vi "GetFeaturesForMCSA(60s).vi"(6 "supported features":string[](array[string]), 8 "error in (no error)":errorcluster, 9 "Metric Cache":variant, 11 "ChannelModel":T4) -> (0 "error out":errorcluster, 2 "channels":T1)   [LabVIEW 2017, in "McsaAnalysisFunctions.lvlib"]
uses:
  <vilib>/addons/InsightCM/Utilities/Analysis/MCSA/McsaAnalysisFunctions.lvlib
  <vilib>/addons/InsightCM/MessageBus/Base/controls/R2_Channel.ctl
  <vilib>/addons/InsightCM/MessageBus/Base/controls/KeyValuePair.ctl
  <vilib>/addons/InsightCM/MessageBus/Base/controls/Metric.ctl
  <vilib>/addons/InsightCM/Utilities/Analysis/MCSA/controls/McsaLowUpdateChannel.ctl
  <vilib>/addons/InsightCM/Utilities/Analysis/Shared/controls/Feature.ctl
  <vilib>/addons/InsightCM/Utilities/Analysis/Shared/controls/AmplitudeScale.ctl
  <vilib>/addons/InsightCM/Utilities/Analysis/Shared/AnalysisHelper.lvlib
  <vilib>/addons/InsightCM/Utilities/Tdms/Tdms.lvlib
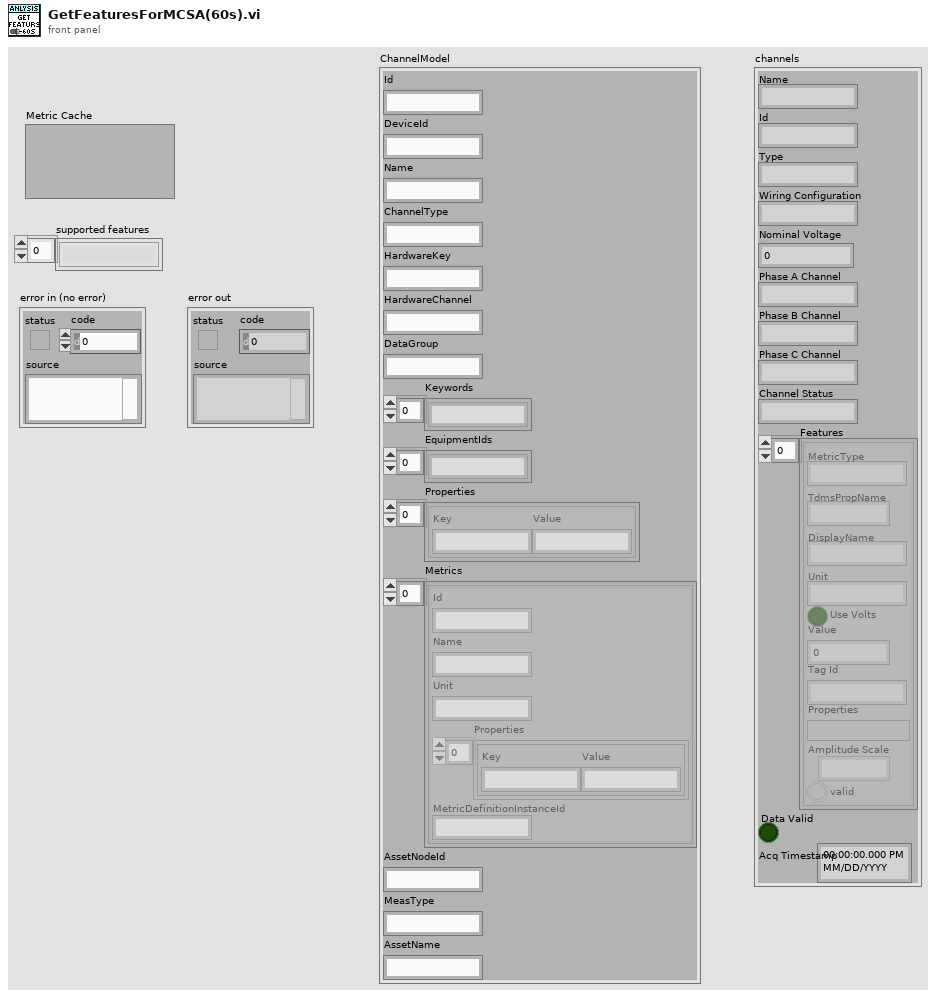
[diagram p1: front panel]
types:
  T1 = typedef "McsaAnalysisFunctions.lvlib/McsaLowUpdateChannel.ctl" = cluster{"Name":string, "Id":string, "Type":string, "Wiring Configuration":string, "Nominal Voltage":dbl, "Phase A Channel":string, "Phase B Channel":string, "Phase C Channel":string, "Channel Status":string, "Features":T2[], "Data Valid":bool, "Acq Timestamp":timestamp}
  T2 = typedef "AnalysisHelper.lvlib/Feature.ctl" = cluster{"MetricType":string, "TdmsPropName":string, "DisplayName":string, "Unit":string, "Use Volts":bool, "Value":dbl, "Tag Id":string, "Properties":variant, "Amplitude Scale":T3, "valid":bool}
  T3 = typedef "AnalysisHelper.lvlib/AmplitudeScale.ctl" = enum16{"rms", "peak", "pk-pk"}
  T4 = typedef "R2_Channel.ctl" = cluster{"Id":string, "DeviceId":string, "Name":string, "ChannelType":string, "HardwareKey":string, "HardwareChannel":string, "DataGroup":string, "Keywords":string[], "EquipmentIds":string[], "Properties":T5[], "Metrics":T6[], "AssetNodeId":string, "MeasType":string, "AssetName":string}
  T5 = typedef "KeyValuePair.ctl" = cluster{"Key":string, "Value":string}
  T6 = typedef "Metric.ctl" = cluster{"Id":string, "Name":string, "Unit":string, "Properties":T5[], "MetricDefinitionInstanceId":string}
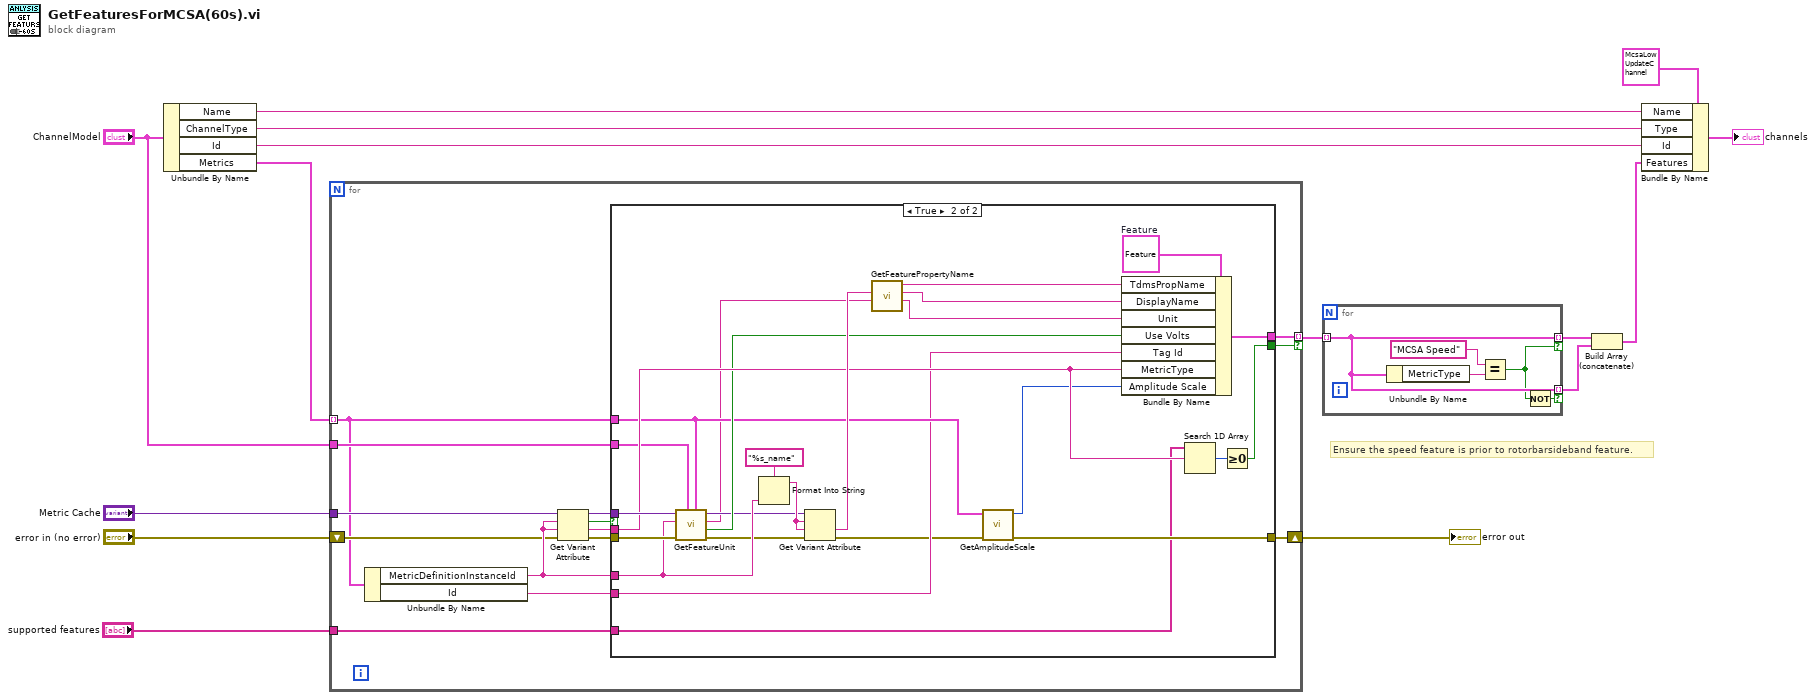
[diagram p0: block diagram]
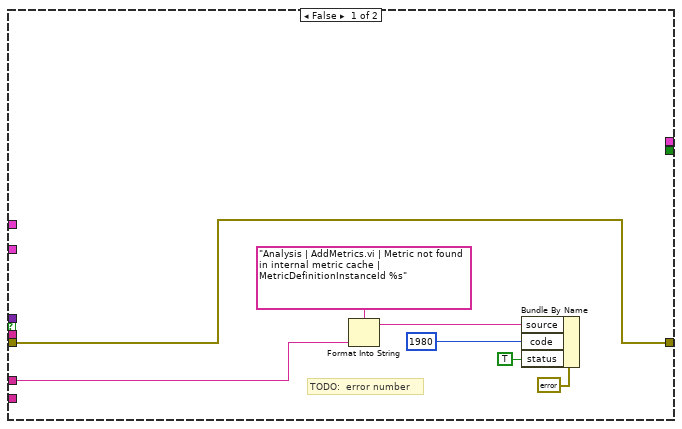
[diagram p2: hidden frame]
diagram:
  # "Ensure the speed feature is prior to rotorbarsideband feature."
  n1 = Unbundle By Name("ChannelModel") -> ("Name"=w7:string, "ChannelType"=w11:string, "Id"=w12:string, "Metrics"=w13:T6[])
  n2 = for {
    tunnel: "Metric Cache" -> [w19]
    tunnel: w13 -> [w17] mode=indexing
    tunnel: [w24] -> w2 mode=indexing if=w23
    shift-right: [w25] -> w9
    shift-left: "error in (no error)" -> [w20]
    tunnel: "ChannelModel" -> [w18]
    tunnel: "supported features" -> [w16]
    n3 = Unbundle By Name(w17) -> ("MetricDefinitionInstanceId"=w21:string, "Id"=w22:string)
    n4 = Get Variant Attribute(Variant=w19, name=w21, default value (empty Variant)=w21, error in=w20) -> (duplicate Variant=w26:variant, found=w27:bool, value=w29:string, error out=w28:errorcluster)
    n5 = case shown="True" w27 {
      tunnel: w28 -> [w30 w54]
      tunnel: w29 -> [_ w52]
      tunnel: w22 -> [_ w38]
      tunnel: w26 -> [_ w53]
      tunnel: [w30 w44] -> w25
      tunnel: [_ w58] -> w24
      tunnel: [_ w50] -> w23
      tunnel: w21 -> [w31 w49]
      tunnel: w17 -> [_ w43]
      tunnel: w18 -> [_ w48]
      tunnel: w16 -> [_ w39]
      frame False {
        # "TODO:  error number"
        n6 = Format Into String(format string="Analysis | AddMetrics.vi | Metric not found in internal metric cache | MetricDefinitionInstanceId %s" ("source"), w31) -> (resulting string=w34:string)  [unwired: 2 in, 1 out]
        n7 = Bundle By Name(cluster=errorcluster {"status"=FALSE, "code"=0, "source"=""} ("error out"), "source"=w34, "code"=1980, "status"=TRUE) -> ()  [unwired: 1 out]
      }
      frame True {
        w61 = T2 {"MetricType"="", "TdmsPropName"="", "DisplayName"="", "Unit"="", "Use Volts"=FALSE, "Value"=0.0, "Tag Id"="", "Properties"=variant(string ""), "Amplitude Scale"=enum."rms", "valid"=FALSE}  # Feature
        n8 = call <vilib>:"GetFeatureUnit.vi"("metric"=w43, "channel"=w48, "error in (no error)"=w54, "metric definitionInstance id"=w49, "metric cache in"=w53) -> ("error out"=w45:errorcluster, "use volts"=w47:bool, "unit"=w41:string, "metric cache out"=w46:variant)  [unwired: 3 in]
        n9 = Format Into String(format string="%s_name", w49) -> (resulting string=w59:string)  [unwired: 2 in, 1 out]
        n10 = Get Variant Attribute(Variant=w46, name=w59, default value (empty Variant)=w59, error in=w45) -> (value=w56:string, error out=w37:errorcluster)  [unwired: 2 out]
        n11 = call <vilib>:"GetFeaturePropertyName.vi"("unit"=w41, "metric name"=w56) -> ("tdms unit value"=w40:string, "display name"=w57:string, "tdms property name"=w55:string)  [unwired: 7 in]
        n12 = call <vilib>:"GetAmplitudeScale.vi"("error in (no error)"=w37, "metric"=w43) -> ("error out"=w44:errorcluster, "amplitude scale"=w42:T3)  [unwired: 8 in]
        n13 = Bundle By Name(cluster=w61, "TdmsPropName"=w55, "DisplayName"=w57, "Unit"=w40, "Use Volts"=w47, "Tag Id"=w38, "MetricType"=w52, "Amplitude Scale"=w42) -> (w58:T2)
        n14 = Search 1D Array(1D array=w39, element=w52) -> (index of element=w51:i32)  [unwired: 1 in]
        n15 = Greater Or Equal To 0?(x=w51) -> (x >= 0?=w50:bool)
      }
    }
  }
  "error out" <- w9
  n16 = for {
    tunnel: w2 -> [w66] mode=indexing
    tunnel: [w66] -> w4 mode=indexing if=w62
    tunnel: [w66] -> w3 mode=indexing if=w65
    n17 = Unbundle By Name(w66) -> ("MetricType"=w64:string)
    n18 = Equal?(x="MCSA Speed", y=w64) -> (x = y?=w62:bool)
    n19 = Not(x=w62) -> (.not. x?=w65:bool)
  }
  n20 = Build Array (concatenate)(w4, w3) -> (w1:T2[])
  n21 = Bundle By Name(cluster=T1 {"Name"="", "Id"="", "Type"="", "Wiring Configuration"="", "Nominal Voltage"=0.0, "Phase A Channel"="", "Phase B Channel"="", "Phase C Channel"="", "Channel Status"="", "Features"=[], "Data Valid"=FALSE, "Acq Timestamp"=timestamp(0 s since 1904-01-01)} ("output cluster"), "Name"=w7, "Type"=w11, "Id"=w12, "Features"=w1) -> (→"channels":T1)
